vi "working_gyro2.vi"(10 "Parâmetros Iniciais":T1={"Gyro Port"=0, "Sensor - Left"=3, "Sensor - Right"=2, "     Color \nSensor Port"=1, "Kp Front"=0.5, "Motor speed"=-15, "Distance to street"=15.0, "Motor speed turns"=16, "Kp Curvas"=0.3} {"Kp Front" format="%.3f"; "Color \nSensor Port" items=["Port 1", "Port 2", "Port 3", "Port 4"]; "Sensor - Right" items=["Port 1", "Port 2", "Port 3", "Port 4"]; "Sensor - Left" items=["Port 1", "Port 2", "Port 3", "Port 4"]; "Gyro Port" items=["Port 1", "Port 2", "Port 3", "Port 4"]}, 11 "NXT/EV3":T3) -> (0 "NXT/EV3 2":T3)   [LabVIEW 2016]
uses:
  <vilib>/NXT/Subs/LVHSConnector.ctl
  <vilib>/NXT/LegoClasses/BrickReference/BrickReference.lvclass
  parametros.ctl
  <vilib>/NXT/Block Support/NXT_InputPort.ctl
  <vilib>/NXT/Block Support/NXT_OutputPort.ctl
  <vilib>/NXT/Dual Mode Library/Display/clearDisplay.vi
  <vilib>/NXT/NXTIO Xnodes/NXTIONodeSubVIs/NXTMoveMotors.vi
  <vilib>/NXT/Dual Mode Library/Display/drawText_Center.vi
  <vilib>/NXT/Dual Mode Library/Sensors/EV3_Gyro_Reset.vi
  <vilib>/NXT/Dual Mode Library/Sensors/EV3_Gyro_Rate.vi
  <vilib>/NXT/Dual Mode Library/Sensors/EV3_Gyro_Angle.vi
  <vilib>/NXT/NXTIO Xnodes/AddressXNode/NXTIOAddress.xnode
  <vilib>/NXT/NXTIO Xnodes/NXTIOXNode/NXTIO.xnode
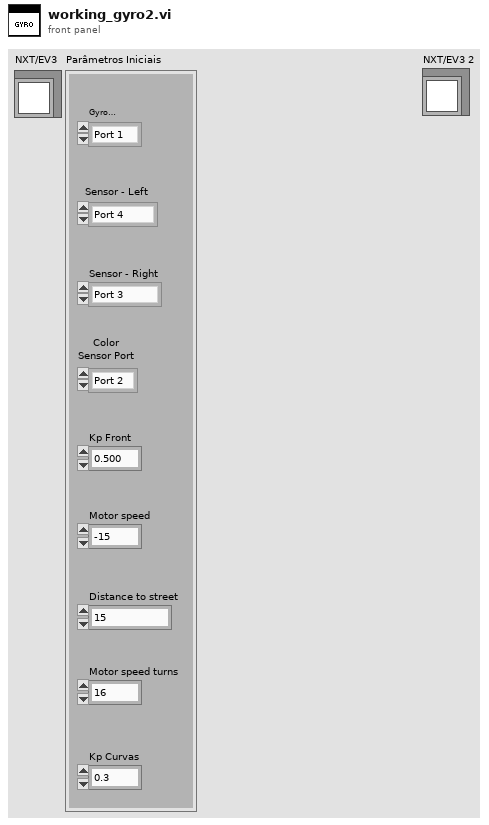
[diagram p1: front panel]
types:
  T1 = typedef "parametros.ctl" = cluster{"Gyro Port":T2, "Sensor - Left":T2, "Sensor - Right":T2, "     Color \nSensor Port":T2, "Kp Front":dbl, "Motor speed":i32, "Distance to street":dbl, "Motor speed turns":i32, "Kp Curvas":dbl}
  T2 = typedef "NXT_InputPort.ctl" = u32
  T3 = typedef "LVHSConnector.ctl" = refnum<class "BrickReference.lvclass">
  T4 = typedef "NXT_OutputPort.ctl" = u8
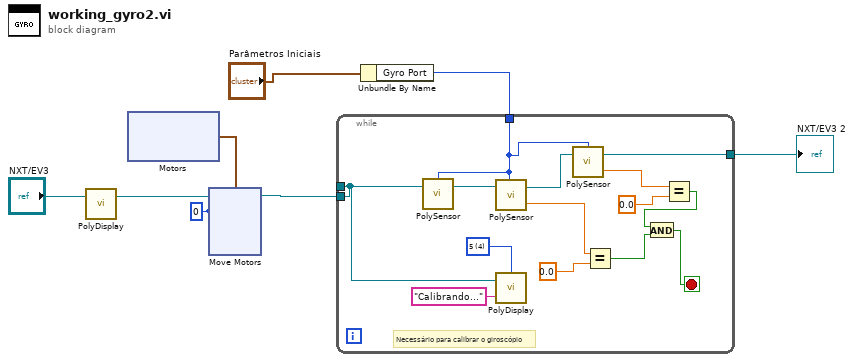
[diagram p0: block diagram]
diagram:
  w1 = i8 0 ("Power/Speed 1")
  n1 = call-poly <vilib>:"PolyDisplay.vi"("NXT/EV3"="NXT/EV3") -> ("NXT/EV3"=w3:T3)  [unwired: 3 in]
  n2 = xnode "Motors"() -> ("Motor"=w4:cluster{"Port":T4, "Port":T4})
  n3 = xnode "Move Motors"("Power/Speed 2"=w1, "Power/Speed 1"=w1, "Motors"=w4, "NXT/EV3"=w3) -> ("NXT/EV3"=w2:T3)
  n4 = Unbundle By Name("Parâmetros Iniciais") -> ("Gyro Port"=w5:T2)
  n5 = while {
    tunnel: w5 -> [w10]
    tunnel: [w9] -> _
    tunnel: [w13] -> w7
    tunnel: w2 -> [w9]
    stop <- w15 stop-if-true
    w11 = i16 4 items=["1", "2", "3", "4", "5", "6", "7", "8", "9", "10", "11", "12"] ("Line")
    # "Necessário para calibrar o giroscópio"
    n6 = call-poly <vilib>:"PolySensor.vi"("NXT/EV3"=w9, "Port (Port 1)"=w10) -> ("NXT/EV3"=w21:T3)  [unwired: 2 in]
    n7 = call-poly <vilib>:"PolySensor.vi"("NXT/EV3"=w21, "Port (Port 1)"=w10) -> ("Degrees/Second"=w20:sgl, "NXT/EV3"=w14:T3)  [unwired: 1 in]
    n8 = call-poly <vilib>:"PolyDisplay.vi"("Text"="Calibrando...", "NXT/EV3"=w9, "Line"=w11) -> ()  [unwired: 1 in, 1 out]
    n9 = call-poly <vilib>:"PolySensor.vi"("NXT/EV3"=w14, "Port (Port 1)"=w10) -> ("Degrees"=w17:sgl, "NXT/EV3"=w13:T3)  [unwired: 1 in]
    n10 = Equal?(x=w20, y=sgl 0.0) -> (x = y?=w19:bool)
    n11 = Equal?(x=w17, y=sgl 0.0) -> (x = y?=w16:bool)
    n12 = And(x=w16, y=w19) -> (x .and. y?=w15:bool)
  }
  "NXT/EV3 2" <- w7
